vi "Win Level.vi"(10 "icon strength":dbl) -> (2 "String":string)   [LabVIEW 2025]
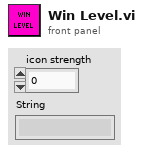
[diagram p1: front panel]
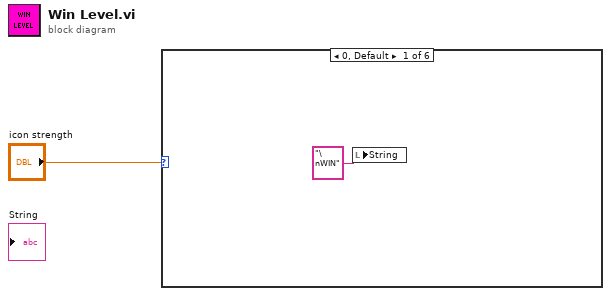
[diagram p0: block diagram]
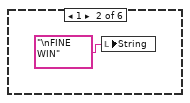
[diagram p2: hidden frame]
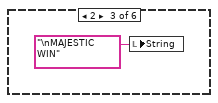
[diagram p3: hidden frame]
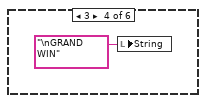
[diagram p4: hidden frame]
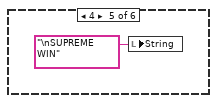
[diagram p5: hidden frame]
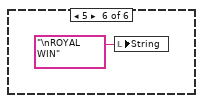
[diagram p6: hidden frame]
diagram:
  n1 = case shown="0, Default" "icon strength" {
    frame 0, Default {
      n2 = local write "String"("\nWIN" ("String")) -> ()
    }
    frame 1 {
      n3 = local write "String"("\nFINE WIN" ("String")) -> ()
    }
    frame 2 {
      n4 = local write "String"("\nMAJESTIC WIN" ("String")) -> ()
    }
    frame 3 {
      n5 = local write "String"("\nGRAND WIN" ("String")) -> ()
    }
    frame 4 {
      n6 = local write "String"("\nSUPREME WIN" ("String")) -> ()
    }
    frame 5 {
      n7 = local write "String"("\nROYAL WIN" ("String")) -> ()
    }
  }
